vi "HighLvCtrl_Loop_Angles.vi"(8 "error in (no error)":errorcluster, 11 "HighLvClasses":T4={"CAlexVersion"=enum."Mobile", "CAlex2 out"=refnum, "ForceField"=refnum}) -> (0 "error out":errorcluster)   [LabVIEW 2016]
uses:
  TypeDef/HighLvControl Cluster.ctl
  Classes/CAlex2/CAlex2.lvclass
  C:/Users/randh/Desktop/CABLE-LABVIEW/CALEX/CAlex2-controller/Classes/SerialChain/SerialChain.lvclass
  C:/Users/randh/Desktop/CABLE-LABVIEW/CALEX/CAlex2-controller/Classes/SerialChain-Cable/SerialChain-Cable.lvclass
  Classes/ForceField/ForceField.lvclass
  Classes/CAlex2/TypeDef/CAlexVersion.ctl
  <vilib>/Analysis/Matrix/Datatypes/RealMatrix.ctl
  <vilib>/Platform/TimedLoop/XDataNode/timing_clust.ctl
  <vilib>/Platform/TimedLoop/XDataNode/nitl_modes.ctl
  <vilib>/Platform/TimedLoop/XDataNode/wakeup.ctl
  TypeDef/IMU_operation.ctl
  Classes/ForceField/TypeDef/FF_Gains.ctl
  Classes/CAlex2/TypeDef/LowerBodyDim.ctl
  Classes/MotorControl/TypeDef/ControllerMode.ctl
  Classes/ForceField/FF_SetGains.vi
  <vilib>/Platform/TimedLoop/XDataNode/XDataNode.xnode
  <vilib>/Platform/TimedLoop/XDataNode/XDNodeRunTimeDep.lvlib
  Classes/SerialChain/SerialChain.lvclass
  Classes/SerialChain-Cable/SerialChain-Cable.lvclass
  <vilib>/Analysis/NI_AALBase.lvlib
  <vilib>/Analysis/Matrix/NI_Matrix.lvlib
  <vilib>/AuZn/auzn custom VIs/AuZnCustomVI.lvlib
  <vilib>/Analysis/baseanly.llb/A x Vector.vi
panel:
  in  "Use Vicon2JointAngle2 ?":bool=TRUE
  in  "Use IMU2JointAngle2 ?":bool=TRUE
  in  "history length (50)":i32=50
  in  "LP":bool=TRUE
  out "QPSolved":bool
  out "Torque Error":dbl[](array[numeric]) format="%#.4f"
  out "Torque":T1(graph)
  out "Joint Angles (deg)":T2(graph)
  out "Desired Torque":dbl[](array[numeric]) format="%#.4f"
  out "Actual Torque":dbl[](array[numeric]) format="%#.4f"
  in  "LockedJoints":i32[](array[numeric])=[2, 1]
  out "Jacobian for Cables":T3 format="%#.3f"
  in  "TargetF(N)":dbl=10.0 format="%#_13g"
  in  "LP fc":dbl=4.0 format="%0.3f"
  in  "QPmode":enum16{"tight", "loose", "adv"}(ring)=enum."adv"
  in  "F range":cluster{"Fmin":dbl, "Fmax":dbl}[](array[cluster])=[{"Fmin"=10.0, "Fmax"=80.0}, {"Fmin"=10.0, "Fmax"=80.0}, {"Fmin"=11.0, "Fmax"=80.0}, {"Fmin"=11.0, "Fmax"=80.0}]
  # "In Cable Order, Not Motor Order"
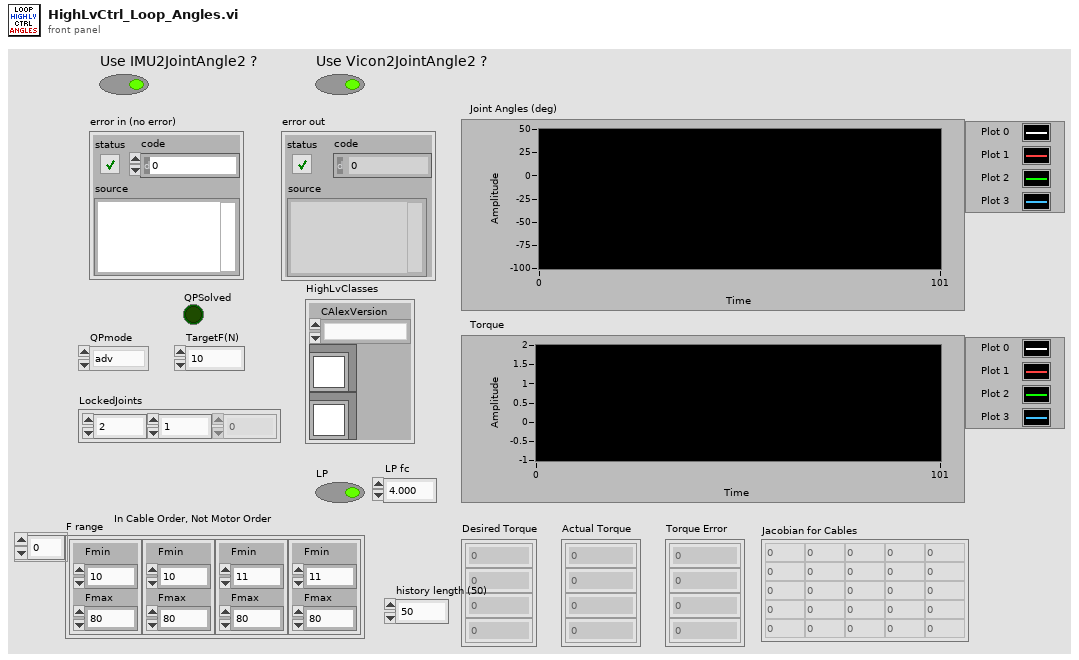
[diagram p1: front panel]
types:
  T1 = cluster{"[0]":dbl, "[1]":dbl, "[2]":dbl, "[3]":dbl, "[4]":dbl, "[5]":dbl, "[6]":dbl, "[7]":dbl, "[8]":dbl}
  T2 = cluster{"Joint Angles (rad)[0]":dbl, "Joint Angles (rad)[1]":dbl, "Joint Angles (rad)[2]":dbl, "Joint Angles (rad)[3]":dbl}
  T3 = typedef "NI_Matrix.lvlib/RealMatrix.ctl" = dbl[][]
  T4 = typedef "HighLvControl Cluster.ctl" = cluster{"CAlexVersion":T5, "CAlex2 out":refnum<class "CAlex2.lvclass">, "ForceField":refnum<class "ForceField.lvclass">}
  T5 = typedef "CAlex2.lvclass/CAlexVersion.ctl" = enum16{"Bilateral_Squat", "Squat", "Treadmill", "Mobile"}
  T6 = typedef "XDNodeRunTimeDep.lvlib/timing_clust.ctl" = cluster{"Expected End [f-1]":u64, "Actual End [f-1]":u64, "Finished Late? [f-1]":bool, "Expected End [i-1]":u64, "Actual End [i-1]":u64, "Finished Late? [i-1]":bool, "Expected Start [i]":u64, "Actual Start [i]":u64, "Expected Start [f]":u64, "Actual Start [f]":u64, "Source Name":string, "Structure Name":string, "Period":i64, "Deadline":i64, "Offset":i64, "Start":i64, "Priority":i32, "Timeout":i32, "Mode":T7, "Wakeup Reason":T8, "Error":errorcluster, "Source Type":string, "Secondary Source Type":string, "Global End Time":u64, "Global Start Time":u64, "Frame Duration":u64, "Iteration Duration":u64, "Assigned CPU":i32, "I/O Scan Engine Mode":u32}
  T7 = typedef "XDNodeRunTimeDep.lvlib/nitl_modes.ctl" = enum32{"No Change", "Process missed periods, maintain original phase", "Discard missed periods, maintain original phase", "Process missed periods, ignore original phase", "Discard missed periods, ignore original phase"}
  T8 = typedef "XDNodeRunTimeDep.lvlib/wakeup.ctl" = enum32{"Normal", "Aborted", "Asynchronous wakeup", "Timing source error", "Timed loop error", "Timeout"}
  T9 = typedef "IMU_operation.ctl" = enum16{"GetData", "ClearStandPos", "SetStandPos"}
  T10 = typedef "CAlex2.lvclass/LowerBodyDim.ctl" = cluster{"BodyDim":cluster{"ThighLt (m)":dbl, "ShankLt (m)":dbl, "HipWd (m)":dbl}, "BodyWt":cluster{"Thigh (kg)":dbl, "Shank (kg)":dbl}, "Cuff Loc":cluster{"HipCuffWd (m)":dbl, "HipCuffHt (m)":dbl, "HipFwdShift (m)":dbl, "ThighToKnee (m)":dbl, "ThighCuffDist (m)":dbl, "ShankToKnee (m)":dbl}}
  T11 = typedef "ForceField.lvclass/FF_Gains.ctl" = cluster{"Kn":dbl, "Dn":dbl, "Kt":dbl, "Dt":dbl, "Kd":dbl, "Ns":dbl}
  T12 = typedef "SerialChain.lvclass/PointOnBody.ctl" = cluster{"Coord4":dbl[], "ID":i32}
  T13 = typedef "MotorControl.lvclass/ControllerMode.ctl" = enum16{"Idle", "FF", "PID"}
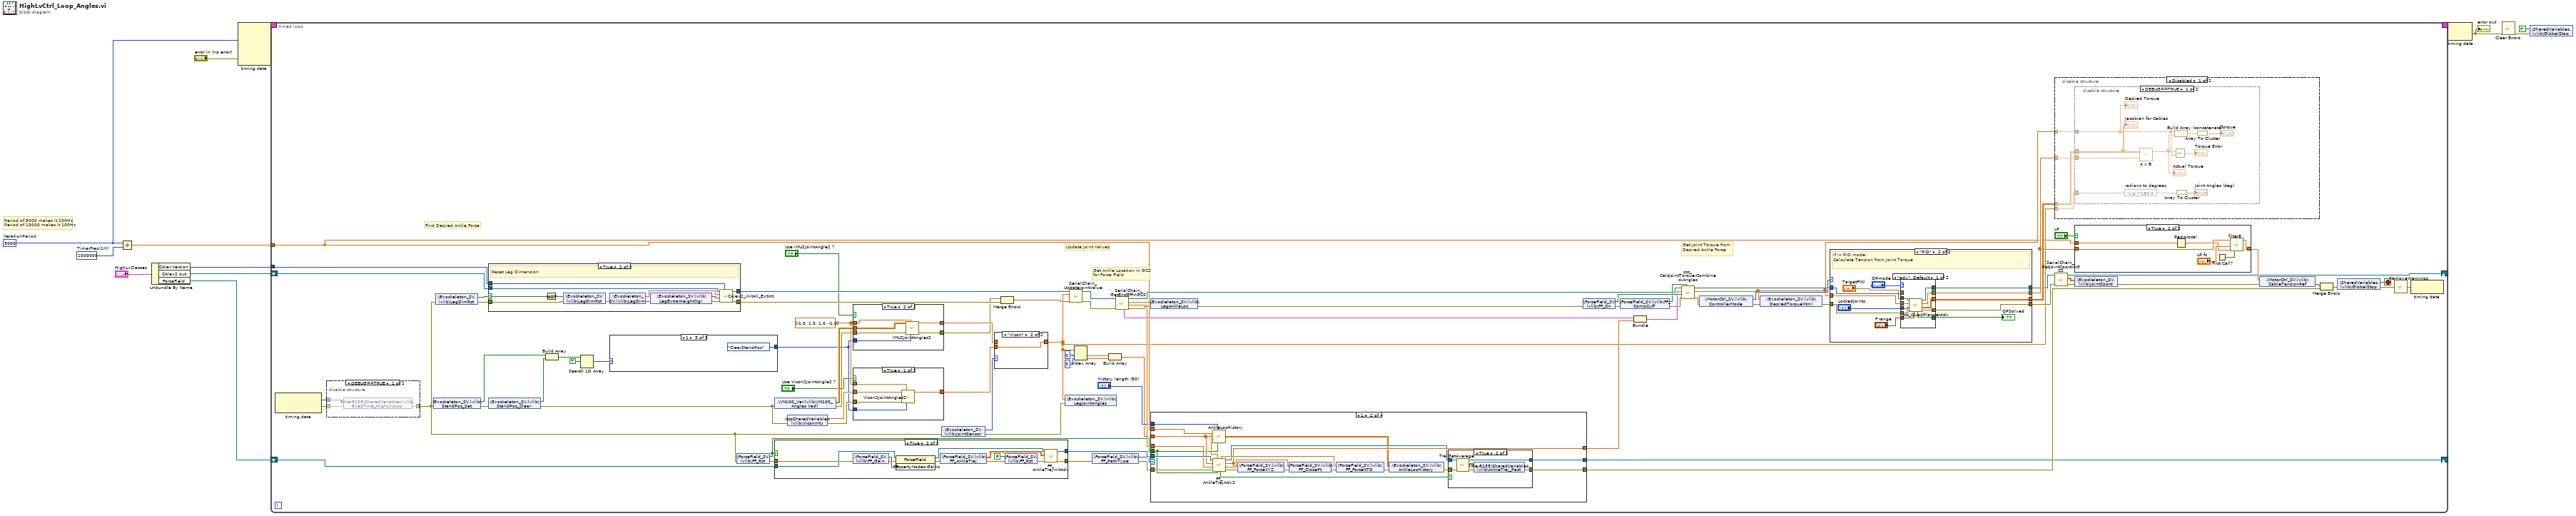
[diagram p0: block diagram]
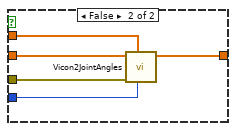
[diagram p5: hidden frame]
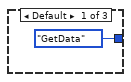
[diagram p6: hidden frame]
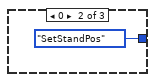
[diagram p7: hidden frame]
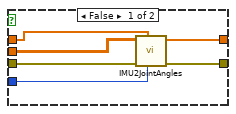
[diagram p8: hidden frame]
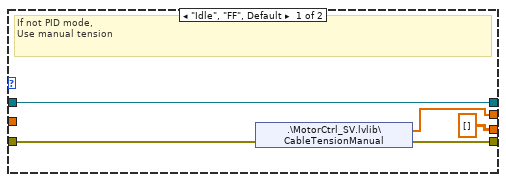
[diagram p11: hidden frame]
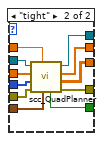
[diagram p12: hidden frame]
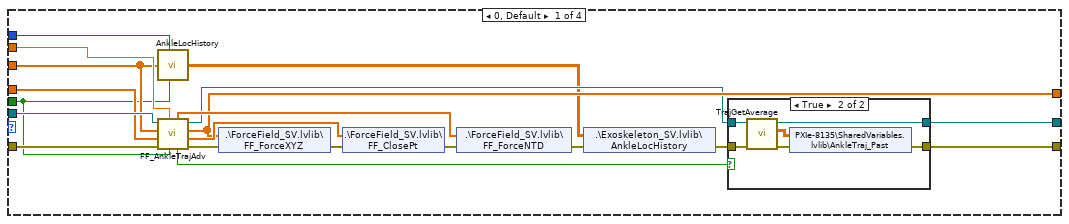
[diagram p15: hidden frame]
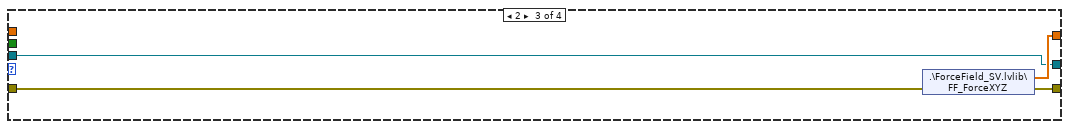
[diagram p18: hidden frame]
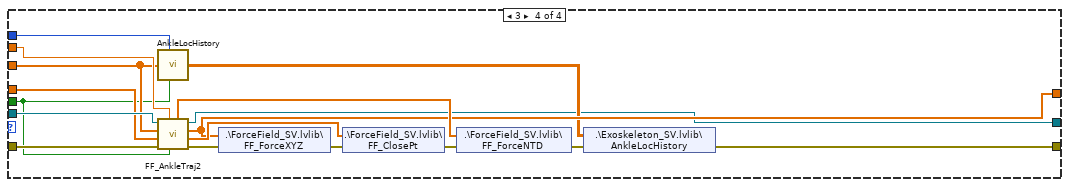
[diagram p19: hidden frame]
diagram:
  w3 = i64 1000000  # TimerFreq(1M)
  w4 = i64 5000  # IterationPeriod
  # "Period of 5000 makes it 200Hz\nPeriod of 10000 makes it 100Hz"
  n1 = Divide(x=w4, y=w3) -> (x/y=w2:dbl)
  n2 = Unbundle By Name("HighLvClasses") -> ("CAlexVersion"=w1:T5, "CAlex2 out"=w9:refnum<class "CAlex2.lvclass">, "ForceField"=w8:refnum<class "ForceField.lvclass">)
  n3 = node-c288(w4, "error in (no error)") -> (w13:T6)  [unwired: 3 in]
  n4 = timed-loop {
    timing: w13 -> [_]
    timing-out: [_] -> w12
    shift-right: [w52] -> _
    shift-left: w9 -> [w95]
    shift-right: [w65] -> _
    shift-left: w8 -> [w92]
    tunnel: w2 -> [w21]
    tunnel: w1 -> [w20]
    stop <- w67 stop-if-true
    w38 = dbl[] [-1.0, 1.0, 1.0, -1.0]
    # "Get Joint Torque from Desired Ankle Force"
    # "Find Desired Ankle Force"
    # "Get Ankle Location in GCS for Force Field"
    # "Update Joint Values"
    n5 = node-c288() -> (w94:i64, w93:errorcluster)  [unwired: 1 in]
    n6 = disable-structure shown="DEBUG==TRUE" {
      disable-tunnel: w94 -> [w146 _]
      disable-tunnel: w93 -> [w145 w147]
      disable-tunnel: [w144 w147] -> w23
      frame condition #0 {
        n7 = shared-variable "PXIe-8135\\SharedVariables.lvlib\\ExecTime_HighLvLoop"(w146, error in=w145) -> (error out=w144:errorcluster)
      }
      frame condition #1 (active) {
      }
    }
    n8 = shared-variable ".\\Exoskeleton_SV.lvlib\\StandPos_Set"(error in=w23) -> (w31:bool, error out=w69:errorcluster)
    n9 = shared-variable ".\\Exoskeleton_SV.lvlib\\LegDimRst"(error in=w23) -> (w76:bool, error out=w87:errorcluster)
    n10 = case shown="True" w76 {
      selector: w76 -> [_ w208]
      tunnel: w95 -> [w201 w213]
      tunnel: [w201 w212] -> w88
      tunnel: w87 -> [w200 w211]
      tunnel: [w200 w206] -> w44
      tunnel: w20 -> [_ w202]
      frame False {
      }
      frame True {
        # "Reset Leg Dimension"
        n11 = Not(x=w208) -> (.not. x?=w209:bool)
        n12 = shared-variable ".\\Exoskeleton_SV.lvlib\\LegDimRst"(w209, error in=w211) -> (error out=w205:errorcluster)
        n13 = shared-variable ".\\Exoskeleton_SV.lvlib\\LegDim"(error in=w205) -> (w210:T10, error out=w204:errorcluster)
        n14 = shared-variable ".\\Exoskeleton_SV.lvlib\\LegExtraWeight(kg)"(error in=w204) -> (w207:cluster{"Thigh":dbl, "Shank":dbl}, error out=w203:errorcluster)
        n15 = call "CAlex2_InitAll_ExtWt.vi"("CAlexVersion"=w202, "error in (no error)"=w203, "ExtraWeight(kg)"=w207, "LegProperties"=w210, "CAlex2 in"=w213) -> ("error out"=w206:errorcluster, "CAlex2 out"=w212:refnum<class "CAlex2.lvclass">)  [unwired: 5 in]
      }
    }
    n16 = shared-variable ".\\Exoskeleton_SV.lvlib\\StandPos_Clear"(error in=w69) -> (w30:bool, error out=w37:errorcluster)
    n17 = Build Array(w31, w30) -> (w29:bool[])
    n18 = Search 1D Array(1D array=w29, element=TRUE) -> (index of element=w28:i32)  [unwired: 1 in]
    n19 = case shown="1" w28 {
      tunnel: [IMU_operation."GetData" ("Operation(GetData)") IMU_operation."SetStandPos" ("Operation(GetData)") IMU_operation."ClearStandPos" ("Operation(GetData)")] -> w26
      frame Default {
      }
      frame 0 {
      }
      frame 1 {
      }
    }
    n20 = shared-variable ".\\ForceField_SV.lvlib\\FF_Rst"(error in=w23) -> (w73:bool, error out=w72:errorcluster)
    n21 = shared-variable ".\\VN100_Var.lvlib\\VN100_Angles (rad)"(error in=w37) -> (w41:dbl[][], error out=w42:errorcluster)
    n22 = case shown="True" w73 {
      tunnel: w92 -> [w187 w199]
      tunnel: [w187 w198] -> w86
      tunnel: w72 -> [w186 w194]
      tunnel: [w186 w188] -> w75
      frame False {
      }
      frame True {
        n23 = shared-variable ".\\ForceField_SV.lvlib\\FF_Gain"(error in=w194) -> (w197:T11, error out=w192:errorcluster)
        n24 = property class="ForceField"(reference=w199, error in=w192, "PropertyNodes:Gains"=w197) -> (reference out=w196:refnum<class "ForceField.lvclass">, error out=w191:errorcluster)
        n25 = shared-variable ".\\ForceField_SV.lvlib\\FF_AnkleTraj"(error in=w191) -> (w195:dbl[][], error out=w190:errorcluster)
        n26 = shared-variable ".\\ForceField_SV.lvlib\\FF_Rst"(FALSE ("FFRst"), error in=w190) -> (error out=w189:errorcluster)
        n27 = call "FF_AnkleTrajInitAdv.vi"("error in (no error)"=w189, "AnkleTraj"=w195, "Force Field Controller in"=w196) -> ("error out"=w188:errorcluster, "Force Field Controller out"=w198:refnum<class "ForceField.lvclass">)  [unwired: 6 in, 1 out]
      }
    }
    n28 = shared-variable ".\\tcpSharedVariables.lvlib\\ViconIMU"(error in=w37) -> (w40:dbl[], error out=w39:errorcluster)
    n29 = case shown="True" "Use IMU2JointAngle2 ?" {
      tunnel: w42 -> [w135 w141]
      tunnel: w41 -> [w134 w140]
      tunnel: w38 -> [w133 w139]
      tunnel: [w132 w138] -> w34
      tunnel: w26 -> [w131 w137]
      tunnel: [w130 w136] -> w25
      frame False {
        n30 = call "IMU2JointAngles.vi"("Operation(GetData)"=w131, "JointAngleDir (-1, 1, 1,-1)"=w133, "error in (no error)"=w135, "IMU in (rad)"=w134) -> ("error out"=w130:errorcluster, "Joint Angles (rad)"=w132:dbl[])  [unwired: 6 in]
      }
      frame True {
        n31 = call "IMU2JointAngles2.vi"("Operation(GetData)"=w137, "JointAngleDir (-1, 1, 1,-1)"=w139, "error in (no error)"=w141, "IMU in (rad)"=w140) -> ("error out"=w136:errorcluster, "Joint Angles (rad)"=w138:dbl[])  [unwired: 6 in]
      }
    }
    n32 = case shown="True" "Use Vicon2JointAngle2 ?" {
      tunnel: w40 -> [w121 w126]
      tunnel: w39 -> [w120 w125]
      tunnel: w38 -> [w119 w124]
      tunnel: [w118 w123] -> w35
      tunnel: w26 -> [w117 w122]
      frame True {
        n33 = call "Vicon2JointAngles2.vi"("Operation(GetData)"=w117, "JointAngleDir([-1,1,1,-1])"=w119, "error in (no error)"=w120, "ViconIMU in (rad)"=w121) -> ("Joint Angles (rad)"=w118:dbl[])  [unwired: 6 in, 1 out]
      }
      frame False {
        n34 = call "Vicon2JointAngles.vi"("Operation(GetData)"=w122, "JointAngleDir([-1,1,1,-1])"=w124, "error in (no error)"=w125, "ViconIMU in (rad)"=w126) -> ("Joint Angles (rad)"=w123:dbl[])  [unwired: 6 in, 1 out]
      }
    }
    n35 = shared-variable ".\\Exoskeleton_SV.lvlib\\JointSensor"(error in=w23) -> (w36:enum16{"IMU", "Vicon"}, error out=w33:errorcluster)
    n36 = case shown="\"Vicon\"" w36 {
      tunnel: w35 -> [_ w143]
      tunnel: [w142 w143] -> w19
      tunnel: w34 -> [w142 _]
      frame "IMU", Default {
      }
      frame "Vicon" {
      }
    }
    n37 = Merge Errors(w25, w44) -> (w43:errorcluster)
    n38 = shared-variable ".\\Exoskeleton_SV.lvlib\\LegJointAngles"(w19, error in=w33) -> ()  [unwired: 1 out]
    n39 = call "SerialChain_UpdateJointValue.vi"("error in (no error)"=w43, "JointAngle (rad | m)"=w19, "SerialChain in"=w88) -> ("error out"=w55:errorcluster, "SerialChain out"=w56:refnum<class "CAlex2.lvclass">)  [unwired: 7 in]
    n40 = Index Array(array=w19, index #1=0 ("index"), index #2=3 ("index")) -> (element #1=w16:dbl, element #2=w15:dbl)
    n41 = shared-variable ".\\ForceField_SV.lvlib\\FF_PathType"(error in=w75) -> (w82:i8, error out=w81:errorcluster)
    n42 = Build Array(w16, w15) -> (w14:dbl[])
    n43 = call "SerialChain_GetEndEffInGCS.vi"("error in (no error)"=w55, "SerialChain in"=w56) -> ("error out"=w74:errorcluster, "Vendeff(GCS)"=w83:dbl[], "Pendeff(GCS)"=w48:dbl[], "SerialChain out"=w90:refnum<class "CAlex2.lvclass">, "EndEffPos"=w91:T12)  [unwired: 5 in]
    n44 = shared-variable ".\\Exoskeleton_SV.lvlib\\LegAnkleLoc"(w48, error in=w74) -> (error out=w79:errorcluster)
    n45 = case shown="1" w82 {
      tunnel: w86 -> [w233 w261 w272 w290]
      tunnel: w81 -> [w229 w257 w271 w286]
      tunnel: [w222 w250 w272 w276] -> w65
      tunnel: [w228 w256 w273 w285] -> w84
      tunnel: w14 -> [w218 w246 _ w279]
      tunnel: w83 -> [w225 w253 _ w282]
      tunnel: w21 -> [w224 w252 _ w281]
      tunnel: w73 -> [w217 w245 _ w278]
      tunnel: [w221 w249 w270 w275] -> w66
      tunnel: "history length (50)" -> [w214 w242 _ w274]
      frame 0, Default {
        n46 = call "AnkleLocHistory.vi"("history length (100)"=w214, "AnkleLoc"=w218, "initialize"=w217) -> ("AnkleLoc"=w219:dbl[][])  [unwired: 2 in]
        n47 = call "FF_AnkleTrajAdv.vi"("Init"=w217, "dt"=w224, "error in (no error)"=w229, "AnkleVelocity"=w225, "AnkleInGCS"=w218, "Force Field Controller in"=w233) -> ("error out"=w227:errorcluster, "ClosestPoint"=w231:dbl[], "ForceXYZ"=w228:dbl[], "Force Field Controller out"=w223:refnum<class "ForceField.lvclass">, "UpdateTrajPrev"=w220:bool, "ForceNTD"=w232:dbl[])
        n48 = shared-variable ".\\ForceField_SV.lvlib\\FF_ForceXYZ"(w228, error in=w227) -> (error out=w226:errorcluster)
        n49 = shared-variable ".\\ForceField_SV.lvlib\\FF_ClosePt"(w231, error in=w226) -> (error out=w230:errorcluster)
        n50 = shared-variable ".\\ForceField_SV.lvlib\\FF_ForceNTD"(w232, error in=w230) -> (error out=w216:errorcluster)
        n51 = shared-variable ".\\Exoskeleton_SV.lvlib\\AnkleLocHistory"(w219, error in=w216) -> (error out=w215:errorcluster)
        n52 = case shown="True" w220 {
          tunnel: w223 -> [w235 w240]
          tunnel: [w235 w241] -> w222
          tunnel: w215 -> [w234 w238]
          tunnel: [w234 w236] -> w221
          frame False {
          }
          frame True {
            n53 = call-dynamic "TrajGetAverage.vi"("error in (no error)"=w238, "ForceField in"=w240) -> ("error out"=w237:errorcluster, "Ankle Traj Ave"=w239:dbl[][], "ForceField out"=w241:refnum<class "ForceField.lvclass">)  [unwired: 7 in]
            n54 = shared-variable "PXIe-8135\\SharedVariables.lvlib\\AnkleTraj_Past"(w239, error in=w237) -> (error out=w236:errorcluster)
          }
        }
      }
      frame 1 {
        n55 = call "AnkleLocHistory.vi"("history length (100)"=w242, "AnkleLoc"=w246, "initialize"=w245) -> ("AnkleLoc"=w247:dbl[][])  [unwired: 2 in]
        n56 = call "FF_AnkleTrajAdv2.vi"("Init"=w245, "dt"=w252, "error in (no error)"=w257, "AnkleVelocity"=w253, "AnkleInGCS"=w246, "Force Field Controller in"=w261) -> ("error out"=w255:errorcluster, "ClosestPoint"=w259:dbl[], "Assistive Force in GCS"=w256:dbl[], "Force Field Controller out"=w251:refnum<class "ForceField.lvclass">, "UpdateTrajAve"=w248:bool, "Assistive Force FnFtFd"=w260:dbl[])
        n57 = shared-variable ".\\ForceField_SV.lvlib\\FF_ForceXYZ"(w256, error in=w255) -> (error out=w254:errorcluster)
        n58 = shared-variable ".\\ForceField_SV.lvlib\\FF_ClosePt"(w259, error in=w254) -> (error out=w258:errorcluster)
        n59 = shared-variable ".\\ForceField_SV.lvlib\\FF_ForceNTD"(w260, error in=w258) -> (error out=w244:errorcluster)
        n60 = shared-variable ".\\Exoskeleton_SV.lvlib\\AnkleLocHistory"(w247, error in=w244) -> (error out=w243:errorcluster)
        n61 = case shown="True" w248 {
          tunnel: w251 -> [w263 w268]
          tunnel: [w263 w269] -> w250
          tunnel: w243 -> [w262 w266]
          tunnel: [w262 w264] -> w249
          frame False {
          }
          frame True {
            n62 = call-dynamic "TrajGetAverage.vi"("error in (no error)"=w266, "ForceField in"=w268) -> ("error out"=w265:errorcluster, "Ankle Traj Ave"=w267:dbl[][], "ForceField out"=w269:refnum<class "ForceField.lvclass">)  [unwired: 7 in]
            n63 = shared-variable "PXIe-8135\\SharedVariables.lvlib\\AnkleTraj_Past"(w267, error in=w265) -> (error out=w264:errorcluster)
          }
        }
      }
      frame 2 {
        n64 = shared-variable ".\\ForceField_SV.lvlib\\FF_ForceXYZ"(error in=w271) -> (w273:dbl[], error out=w270:errorcluster)
      }
      frame 3 {
        n65 = call "AnkleLocHistory.vi"("history length (100)"=w274, "AnkleLoc"=w279, "initialize"=w278) -> ("AnkleLoc"=w280:dbl[][])  [unwired: 2 in]
        n66 = call "FF_AnkleTraj2.vi"("Init"=w278, "dt"=w281, "error in (no error)"=w286, "AnkleVelocity"=w282, "AnkleInGCS"=w279, "Force Field Controller in"=w290) -> ("error out"=w284:errorcluster, "ClosePt"=w288:dbl[], "Force"=w285:dbl[], "Force Field Controller out"=w276:refnum<class "ForceField.lvclass">, "ForceComp"=w289:dbl[])  [unwired: 1 in]
        n67 = shared-variable ".\\ForceField_SV.lvlib\\FF_ForceXYZ"(w285, error in=w284) -> (error out=w283:errorcluster)
        n68 = shared-variable ".\\ForceField_SV.lvlib\\FF_ClosePt"(w288, error in=w283) -> (error out=w287:errorcluster)
        n69 = shared-variable ".\\ForceField_SV.lvlib\\FF_ForceNTD"(w289, error in=w287) -> (error out=w277:errorcluster)
        n70 = shared-variable ".\\Exoskeleton_SV.lvlib\\AnkleLocHistory"(w280, error in=w277) -> (error out=w275:errorcluster)
      }
    }
    n71 = shared-variable ".\\ForceField_SV.lvlib\\FF_On"(error in=w79) -> (w78:bool, error out=w80:errorcluster)
    n72 = shared-variable ".\\ForceField_SV.lvlib\\FF_CompCuff"(error in=w80) -> (w64:bool, error out=w77:errorcluster)
    n73 = Bundle("EndEffPos"=w91, "Force"=w84) -> (w85:cluster{"EndEffPos":T12, "Force":dbl[]})  [unwired: 1 in]
    n74 = call "scc_CalcJointTorque-Combined-Angles.vi"("CuffWtComp?(T)"=w64, "error in (no error)"=w77, "ExternalForce(T)"=w78, "External Force (In GCS)"=w85, "SerialChain_Cable in"=w90) -> ("error out"=w61:errorcluster, "DesiredTorque(Nm)"=w47:dbl[], "SerialChain_Cable out"=w89:refnum<class "CAlex2.lvclass">)  [unwired: 4 in]
    n75 = shared-variable ".\\MotorCtrl_SV.lvlib\\ControllerMode"(error in=w61) -> (w62:T13, error out=w46:errorcluster)
    n76 = shared-variable ".\\Exoskeleton_SV.lvlib\\DesiredTorque(Nm)"(w47, error in=w46) -> (error out=w45:errorcluster)
    n77 = case shown="\"PID\"" w62 {
      tunnel: [w151 w164] -> w54
      tunnel: w45 -> [w150 w163]
      tunnel: w89 -> [w151 w162]
      tunnel: [T3 [] ("Jacobian for Cables") w158] -> w71
      tunnel: w47 -> [_ w157]
      tunnel: [w152 w156] -> w63
      tunnel: [w149 w155] -> w53
      frame "Idle", "FF", Default {
        # "If not PID mode,\nUse manual tension"
        n78 = shared-variable ".\\MotorCtrl_SV.lvlib\\CableTensionManual"(error in=w150) -> (w152:dbl[], error out=w149:errorcluster)
      }
      frame "PID" {
        # "If in PID mode:\nCalculate Tension from Joint Torque"
        n79 = case shown="\"adv\", Default" "QPmode" {
          tunnel: w163 -> [w167 w185]
          tunnel: w162 -> [w173 w184]
          tunnel: w157 -> [w172 w177]
          tunnel: [w174 w183] -> w164
          tunnel: "F range" -> [w169 w182]
          tunnel: [w168 w181] -> w161
          tunnel: [w171 w180] -> w156
          tunnel: [w170 w179] -> w155
          tunnel: "TargetF(N)" -> [_ w178]
          tunnel: "LockedJoints" -> [w166 w176]
          tunnel: [w165 w175] -> w158
          frame "adv", Default {
            n80 = call "scc_QuadPlannerAdv.vi"("F range (of each cable)"=w169, "error in (no error)"=w167, "LockedJoint(StartFrom0)"=w166, "DesireTorque(Nm)"=w172, "SerialChain_Cable in"=w173) -> ("error out"=w170:errorcluster, "Jacobian for Cables"=w165:T3, "Planned Tension"=w171:dbl[], "SerialChain_Cable out"=w174:refnum<class "CAlex2.lvclass">, "Solved"=w168:bool)  [unwired: 2 in]
          }
          frame "tight" {
            n81 = call "scc_QuadPlanner.vi"("F range"=w182, "TargetF(N)"=w178, "error in (no error)"=w185, "LockedJoint(StartFrom0)"=w176, "DesireTorque(Nm)"=w177, "SerialChain_Cable in"=w184) -> ("error out"=w179:errorcluster, "Jacobian for Cables"=w175:T3, "Planned Tension"=w180:dbl[], "SerialChain_Cable out"=w183:refnum<class "CAlex2.lvclass">, "Solved"=w181:bool)  [unwired: 1 in]
          }
        }
        "QPSolved" <- w161
      }
    }
    n82 = disable-structure shown="Disabled" {
      disable-tunnel: w71 -> [w106 _]
      disable-tunnel: w63 -> [w105 _]
      disable-tunnel: w47 -> [w104 _]
      disable-tunnel: w19 -> [w103 _]
      frame Disabled {
        n83 = disable-structure shown="DEBUG==TRUE" {
          disable-tunnel: w106 -> [w116 _]
          disable-tunnel: w105 -> [w115 _]
          disable-tunnel: w103 -> [w114 _]
          disable-tunnel: w104 -> [w108 _]
          frame condition #0 {
            n84 = expression code="(x/pi)*180.0" "radians to degrees"(w114) -> (w111:dbl[])
            n85 = call-poly <vilib>:"A x B.vi"("Vector"=w115, "A"=w116) -> ("A x Vector"=w109:dbl[])  [unwired: 1 out]
            "Actual Torque" <- w109
            n86 = Subtract(x=w109, y=w108) -> (x-y=→"Torque Error":dbl[])
            n87 = Build Array (concatenate)(w108, w109) -> (w112:dbl[])
            n88 = Array To Cluster(array=w111) -> (cluster=→"Joint Angles (deg)":T2)
            n89 = Array To Cluster(array=w112) -> (cluster=→"Torque":T1)
            "Jacobian for Cables" <- w116
            "Desired Torque" <- w108
          }
          frame condition #1 (active) {
          }
        }
      }
      frame Enabled {
      }
    }
    n90 = call "SerialChain_GetJointCoordInGCS.vi"("error in (no error)"=w53, "SerialChain in"=w54) -> ("error out"=w50:errorcluster, "Joint Coord in GCS"=w51:dbl[][], "SerialChain out"=w52:refnum<class "CAlex2.lvclass">)  [unwired: 5 in, 2 out]
    n91 = case shown="True" "LP" {
      tunnel: w63 -> [w96 w100]
      tunnel: [w96 w99] -> w60
      tunnel: w21 -> [_ w97]
      frame False {
      }
      frame True {
        n92 = Reciprocal(x=w97) -> (1/x=w101:dbl)
        n93 = First Call?() -> (First Call?: T/F=w98:bool)
        n94 = call "filter8.vi"("initialize"=w98, "sampling freq: fs"=w101, "low cutoff freq: fl"="LP fc", "X"=w100) -> ("Filtered X"=w99:dbl[])  [unwired: 7 in]
      }
    }
    n95 = shared-variable ".\\Exoskeleton_SV.lvlib\\JointCoord"(w51, error in=w50) -> (error out=w49:errorcluster)
    n96 = shared-variable ".\\MotorCtrl_SV.lvlib\\CableTensionRef"(w60, error in=w49) -> (error out=w70:errorcluster)
    n97 = Merge Errors(w70, w66) -> (w68:errorcluster)
    n98 = shared-variable ".\\SharedVariables.lvlib\\GlobalStop"(error in=w68) -> (w67:bool, error out=w59:errorcluster)
    n99 = call <vilib>:"RemoveWarnings.vi"("error in (no error)"=w59) -> ("error out"=w58:errorcluster)
    n100 = node-c288(w58) -> ()  [unwired: 1 out]
  }
  n101 = node-c288(w12) -> (w6:errorcluster)
  "error out" <- w6
  n102 = call <vilib>:"Clear Errors.vi"("error in (no error)"=w6) -> ("error out"=w5:errorcluster)  [unwired: 5 in, 1 out]
  n103 = shared-variable ".\\SharedVariables.lvlib\\GlobalStop"(TRUE ("GlobalStop"), error in=w5) -> ()  [unwired: 1 out]
